vi "target.vi"() -> ()   [LabVIEW 2020]
uses:
  <vilib>/rvi/interface/RandomDataEmulation/niFpgaRandomDataHandleErrors.vi
  <vilib>/rvi/DataTransferAndStorage/Container/Common/niFpgaContainerExecOnDevCompGetState.vi
  <vilib>/rvi/Emulation/niFpgaEmulationIsFPGAContextNoSignature.vi
  <vilib>/rvi/DataTransferAndStorage/Container/Common/niFpgaContainerGetUniqueNameForEmu.vi
  <vilib>/rvi/Memory/Memory_Emulation/niFpgaMemoryEmulationCacheClearOnFirstRun.vi
  <vilib>/rvi/Memory/Memory_Emulation/nirvimemoryEmulationManagerCache_MakeExclusive.vi
  <vilib>/rvi/Memory/Memory_Emulation/niFpgaMemoryEmulationValidateCache.vi
  <vilib>/rvi/Memory/Memory_Emulation/nirvimemoryEmulationManagerCache_InsertValue.vi
  <vilib>/Utility/error.llb/Clear Errors.vi
  <vilib>/rvi/Memory/Memory_Emulation/nirvimemoryEmulationManagerCache_ReleaseExclusive.vi
  <vilib>/rvi/Memory/Memory_Emulation/nirvimemoryEmulationManagerCache_GetValue.vi
  <vilib>/rvi/Memory/Memory_Emulation/nirvimemoryEmulationManagerCache_SetValue.vi
  <vilib>/rvi/Emulation/niFpgaProcessEmulError.vi
  <vilib>/rvi/Emulation/niFpgaSctlEmulationGetInTimedLoop.vi
  <vilib>/rvi/errors/nirviReportUnexpectedCaseInternalError (U32).vi
  <vilib>/rvi/Emulation/niFpgaSctlEmulationResourceMgr.vi
  <vilib>/rvi/DataTransferAndStorage/Container/XNode/niFpgaContainer.xnode
  <vilib>/rvi/interface/RandomDataEmulation/nirviRandomDataFpgaReadWriteTemplate.vi
  <vilib>/rvi/DataTransferAndStorage/Register/Emulation/niFpgaRegisterEmulationRefIn.vi
  <vilib>/rvi/Memory/Memory_Emulation/niFpgaMemoryEmulationRefIn.vi
panel:
  out "clock ticks":u32
  out "y":fxp<+/-,33,17>
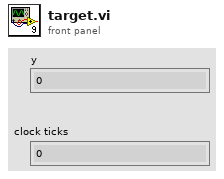
[diagram p1: front panel]
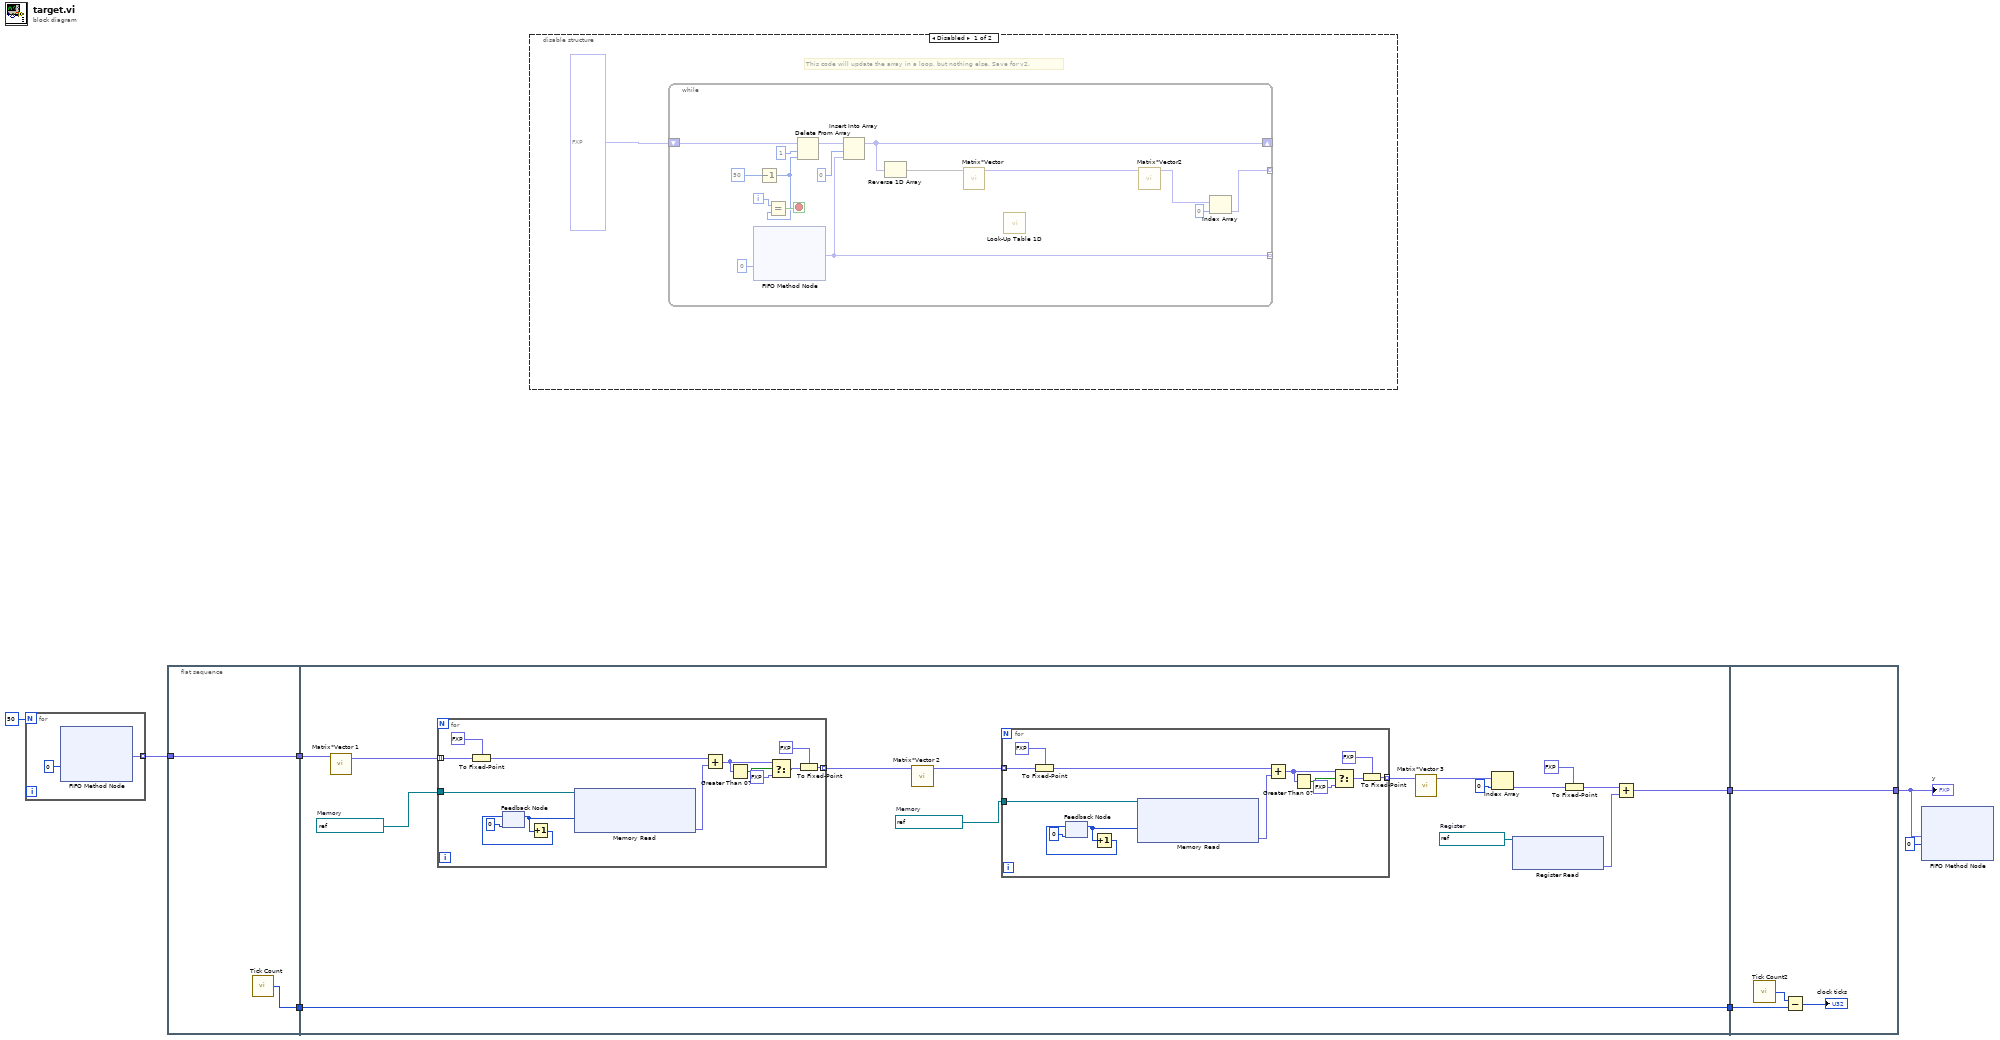
[diagram p0: block diagram]
diagram:
  n1 = for {
    N: 50 -> [_]
    tunnel: [w9] -> w4 mode=indexing
    n2 = xnode ("FIFO Method Node")("Timeout"=0) -> ("Element"=w9:fxp<+/-,32,16>)  [unwired: 1 in, 2 out]
  }
  n3 = flat-sequence {
    tunnel: [w12] -> w8
    tunnel: w4 -> [w11]
    tunnel: [w11] -> w3
    tunnel: w8 -> [w20]
    tunnel: [w20] -> w7
    tunnel: [w19] -> w6
    tunnel: w3 -> [w18]
    tunnel: w7 -> [w59]
    tunnel: w6 -> [w57]
    tunnel: [w57] -> w1
    frame #0 {
      n4 = call "Tick Count"() -> ("Tick Count(Ticks)"=w12:u32)
    }
    frame #1 {
      w14 = refnum<k21> "Memory-B_1"  # Memory
      w17 = refnum<k21> "Memory-B_0"  # Memory
      w24 = refnum<k21> "Register-B_2"  # Register
      n5 = call "Matrix*Vector 1"("Vector b"=w18) -> ("Vector c"=w26:fxp<+/-,32,16>[])  [unwired: 10 in]
      n6 = for {
        tunnel: w26 -> [w48] mode=indexing
        tunnel: [w44] -> w16 mode=indexing
        tunnel: w17 -> [w43]
        n7 = To Fixed-Point(fixed-point type=fxp<+/-,32,16> 0.0 ("f"), number=w48) -> (fixed-point=w52:fxp<+/-,32,16>)
        n8 = feedback #1(u32 0 ("Timeout")) -> (w51:u32)
        n9 = Increment(x=w51) -> (x+1=w50:u32)
        n10 = feedback-in #1(w50) -> ()
        n11 = xnode ("Memory Read")("Address"=w51, "Memory In"=w43) -> ("Data"=w49:fxp<+/-,32,16>)  [unwired: 1 out]
        n12 = Add(x=w52, y=w49) -> (x+y=w54:fxp<+/-,33,17>)
        n13 = Greater Than 0?(x=w54) -> (x > 0?=w56:bool)
        n14 = Select(t=w54, s=w56, f=fxp<+/-,33,17> 0.0) -> (s? t:f=w45:fxp<+/-,33,17>)
        n15 = To Fixed-Point(fixed-point type=fxp<+/-,32,16> 0.0 ("f"), number=w45) -> (fixed-point=w44:fxp<+/-,32,16>)
      }
      n16 = call "Matrix*Vector 2"("Vector b"=w16) -> ("Vector c"=w15:fxp<+/-,32,16>[])  [unwired: 10 in]
      n17 = for {
        tunnel: w15 -> [w34] mode=indexing
        tunnel: [w30] -> w13 mode=indexing
        tunnel: w14 -> [w29]
        n18 = To Fixed-Point(fixed-point type=fxp<+/-,32,16> 0.0 ("f"), number=w34) -> (fixed-point=w38:fxp<+/-,32,16>)
        n19 = feedback #2(u32 0 ("Timeout")) -> (w37:u32)
        n20 = Increment(x=w37) -> (x+1=w36:u32)
        n21 = feedback-in #2(w36) -> ()
        n22 = xnode ("Memory Read")("Address"=w37, "Memory In"=w29) -> ("Data"=w35:fxp<+/-,32,16>)  [unwired: 1 out]
        n23 = Add(x=w38, y=w35) -> (x+y=w40:fxp<+/-,33,17>)
        n24 = Greater Than 0?(x=w40) -> (x > 0?=w42:bool)
        n25 = Select(t=w40, s=w42, f=fxp<+/-,33,17> 0.0) -> (s? t:f=w31:fxp<+/-,33,17>)
        n26 = To Fixed-Point(fixed-point type=fxp<+/-,32,16> 0.0 ("f"), number=w31) -> (fixed-point=w30:fxp<+/-,32,16>)
      }
      n27 = call "Matrix*Vector 3"("Vector b"=w13) -> ("Vector c"=w28:fxp<+/-,64,38>[])  [unwired: 10 in]
      n28 = Index Array(array=w28, index=0) -> (element=w21:fxp<+/-,64,38>)
      n29 = xnode ("Register Read")("Register In"=w24) -> ("Data"=w23:fxp<+/-,32,16>)  [unwired: 1 out]
      n30 = To Fixed-Point(fixed-point type=fxp<+/-,32,16> 0.0 ("f"), number=w21) -> (fixed-point=w25:fxp<+/-,32,16>)
      n31 = Add(x=w25, y=w23) -> (x+y=w19:fxp<+/-,33,17>)
    }
    frame #2 {
      n32 = call "Tick Count2"() -> ("Tick Count(Ticks)"=w60:u32)
      n33 = Subtract(x=w60, y=w59) -> (x-y=→"clock ticks":u32)
    }
  }
  n34 = disable-structure shown="Disabled" {
    frame Disabled {
      # "This code will update the array in a loop, but nothing else. Save for v2."
      n35 = while {
        tunnel: [w75] -> w62 mode=indexing
        shift-right: [w65] -> _
        shift-left: fxp<+/-,32,16>[] [0.0, 0.0, 0.0, 0.0, 0.0, 0.0, 0.0, 0.0, 0.0, 0.0, 0.0, 0.0, 0.0, 0.0, 0.0, 0.0, 0.0, 0.0, 0.0, 0.0, 0.0, 0.0, 0.0, 0.0, 0.0, 0.0, 0.0, 0.0, 0.0, 0.0, 0.0, 0.0, 0.0, 0.0, 0.0, 0.0, 0.0, 0.0, 0.0, 0.0, 0.0, 0.0, 0.0, 0.0, 0.0, 0.0, 0.0, 0.0, 0.0, 0.0] -> [w74]
        tunnel: [w64] -> w61 mode=indexing
        i -> [w78]
        stop <- w77 stop-if-true
        n36 = xnode ("FIFO Method Node")("Timeout"=0) -> ("Element"=w75:fxp<+/-,32,16>)  [unwired: 1 in, 2 out]
        n37 = Decrement(x=u32 50) -> (x-1=w70:u32)
        n38 = Equal?(x=w78, y=w70) -> (x = y?=w77:bool)
        n39 = Delete From Array(array=w74, length=1, index=w70) -> (array with subset deleted=w73:fxp<+/-,32,16>[])  [unwired: 1 out]
        n40 = Insert Into Array(array=w73, index=0, new element=w75) -> (w65:fxp<+/-,32,16>[])
        n41 = Reverse 1D Array(array=w65) -> (reversed array=w69:fxp<+/-,32,16>[])
        n42 = call "Matrix*Vector"("Vector b"=w69) -> ("Vector c"=w68:fxp<+/-,32,16>[])  [unwired: 10 in]
        n43 = call "Look-Up Table 1D"() -> ()  [unwired: 9 in, 1 out]
        n44 = call "Matrix*Vector2"("Vector b"=w68) -> ("Vector c"=w67:fxp<+/-,37,21>[])  [unwired: 10 in]
        n45 = Index Array(array=w67, index=0) -> (element=w64:fxp<+/-,37,21>)
      }
    }
    frame Enabled {
    }
  }
  n46 = xnode ("FIFO Method Node")("Element"=w1, "Timeout"=0) -> ()  [unwired: 1 in, 2 out]
  "y" <- w1
